vi "StaticOn.vi"(7 "LabVIEW Web Service Request":refnum<class "Web Request.lvclass">, 10 "On":u8=1, 11 "DevID":string) -> ()   [LabVIEW 2014]
uses:
  <vilib>/wsapi/Web Request.lvclass
  Controller/Messages/Turn mTEC on/Turn mTEC on.lvclass
  Controller/Messages/Turn mTEC on/Turn mTEC on.lvclass/Turn mTEC on.ctl
  Controller/Messages/Turn mTEC on/Write DevId.vi
  Controller/Messages/Turn mTEC on/Write On.vi
  Controller/Controller.lvclass
panel:
  # "Use the Web Service Request input terminal to call the VIs on the Web Services palette. Do not remove it from the connector pane unless you don't need access to the palette."
  # "Each additional control wired to the connector pane will be available as an input in the URL. To include an indicator in terminal-mode output (the default setting), it must also be wired to the connector pane."
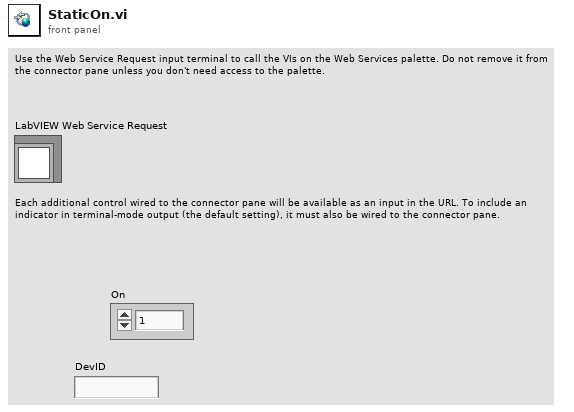
[diagram p1: front panel]
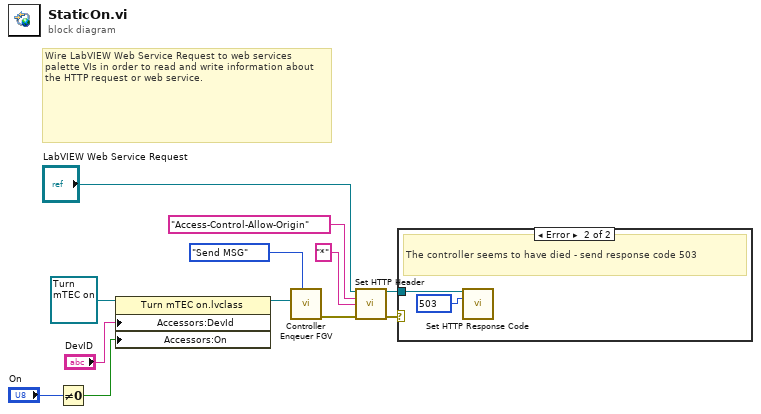
[diagram p0: block diagram]
diagram:
  # "Wire LabVIEW Web Service Request to web services palette VIs in order to read and write information about the HTTP request or web service."
  n1 = Not Equal To 0?(x="On") -> (x != 0?=w2:bool)
  n2 = property class="Turn mTEC on.lvclass"(reference=refnum<class "Turn mTEC on.lvclass"> refnum ("Controller:Turn mTEC on.lvclass"), "Accessors:DevId"="DevID", "Accessors:On"=w2) -> (reference out=w1:refnum<class "Turn mTEC on.lvclass">)  [unwired: 1 in, 1 out]
  n3 = call "Controller Enqeuer FGV.vi"("State"=enum16{"Store", "Send MSG"}."Send MSG", "MSG"=w1) -> ("error out"=w7:errorcluster)  [unwired: 9 in]
  n4 = call <vilib>:"Set HTTP Header.vi"("LabVIEW Web Service Request"="LabVIEW Web Service Request", "header"="Access-Control-Allow-Origin", "header value"="*", "error in (no error)"=w7) -> ("LabVIEW Web Service Request out"=w10:refnum<class "Web Request.lvclass">, "error out"=w9:errorcluster)  [unwired: 10 in]
  n5 = case shown="Error" w9 {
    tunnel: w10 -> [_ w13]
    frame No Error {
    }
    frame Error {
      w14 = 503 items=["100"=100, "101"=101, "200"=200, "201"=201, "202"=202, "203"=203, "204"=204, "205"=205, "206"=206, "300"=300, "301"=301, "302"=302, "303"=303, "304"=304, "305"=305, "306"=306, "307"=307, "400"=400, "401"=401, "402"=402, "403"=403, "404"=404, "405"=405, "406"=406, "407"=407, "408"=408, "409"=409, "410"=410, "411"=411, "412"=412, "413"=413, "414"=414, "415"=415, "416"=416, "417"=417, "500"=500, "501"=501, "502"=502, "503"=503, "504"=504, "505"=505] ("response code (200)")
      # "The controller seems to have died - send response code 503"
      n6 = call <vilib>:"Set HTTP Response Code.vi"("LabVIEW Web Service Request"=w13, "response code (200)"=w14) -> ()  [unwired: 12 in, 2 out]
    }
  }
